vi "Scott -- strain -- manipulate sweep parameters V0.vi"(7 "sweep parameters action":T3, 10 "strain sweep control":T1={"just in case"=TRUE, "Piezo Amplifier settings"={"Gain "=69.44, "offset (V)"=69.44}, "voltage-parameters-IN"={"phase "=2.88, "amplitude (V)"=-0.7854, "offset (V)"=0.28, "time delay (sec)"=0.5, "period (sec)"=50.0, "shape"=enum."triangle"}, "Lockin Settings"=[{"Offset"=FALSE, "GPIB Address"=6}, {"Offset"=TRUE, "GPIB Address"=7}], "VISA address Agilent  IN"="GPIB0::22::INSTR", "number of iterations"=1.0, "Piezo sweep settings"={"max Piezo voltage (V) "=69.44, "min Piezo voltage (V)"=69.44, "delay (sec)"=69.44, "period (sec)"=69.44, "shape"=enum."triangle"}}) -> (2 "strain sweep control OUT":T1={"just in case"=TRUE, "Piezo Amplifier settings"={"Gain "=69.44, "offset (V)"=69.44}, "voltage-parameters-IN"={"phase "=2.88, "amplitude (V)"=-0.7854, "offset (V)"=0.28, "time delay (sec)"=0.5, "period (sec)"=50.0, "shape"=enum."triangle"}, "Lockin Settings"=[{"Offset"=FALSE, "GPIB Address"=6}, {"Offset"=TRUE, "GPIB Address"=7}], "VISA address Agilent  IN"="", "number of iterations"=1.0, "Piezo sweep settings"={"max Piezo voltage (V) "=69.44, "min Piezo voltage (V)"=69.44, "delay (sec)"=69.44, "period (sec)"=69.44, "shape"=enum."triangle"}})   [LabVIEW 2014]
uses:
  Scott -- strain -- strain sweep control.ctl
  FSU/ScottRiggs/Piezo2/voltage-wave-generator-parameters.ctl
  Scott -- strain -- sweep parameter action.ctl
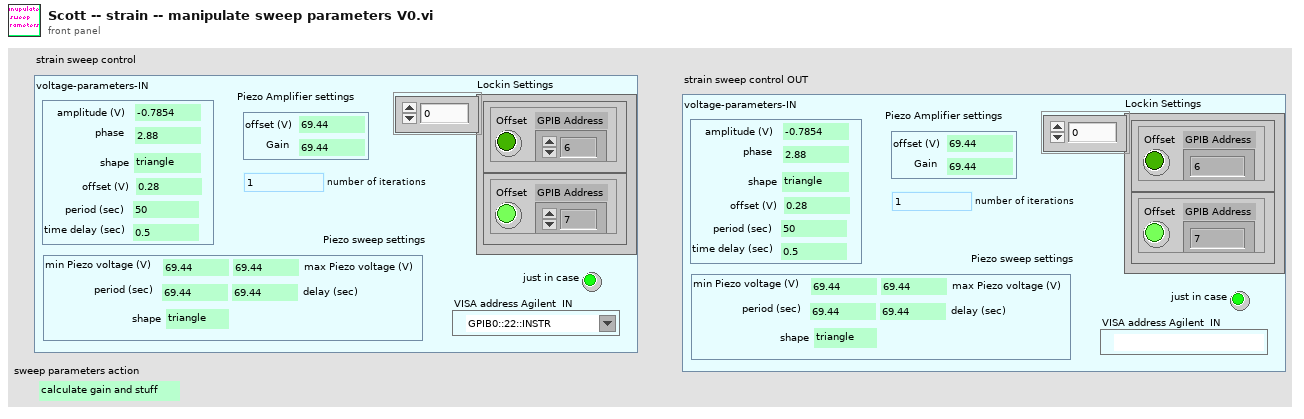
[diagram p1: front panel]
types:
  T1 = typedef "Scott -- strain -- strain sweep control.ctl" = cluster{"just in case":bool, "Piezo Amplifier settings":cluster{"Gain ":dbl, "offset (V)":dbl}, "voltage-parameters-IN":T2, "Lockin Settings":cluster{"Offset":bool, "GPIB Address":i16}[], "VISA address Agilent  IN":refnum<visa-resource-name>, "number of iterations":dbl, "Piezo sweep settings":cluster{"max Piezo voltage (V) ":dbl, "min Piezo voltage (V)":dbl, "delay (sec)":dbl, "period (sec)":dbl, "shape":enum16{"triangle", "sine", "none"}}}
  T2 = typedef "voltage-wave-generator-parameters.ctl" = cluster{"phase ":dbl, "amplitude (V)":dbl, "offset (V)":dbl, "time delay (sec)":dbl, "period (sec)":dbl, "shape":enum16{"triangle", "sine", "none"}}
  T3 = typedef "Scott -- strain -- sweep parameter action.ctl" = enum16{"calculate gain and stuff", "none"}
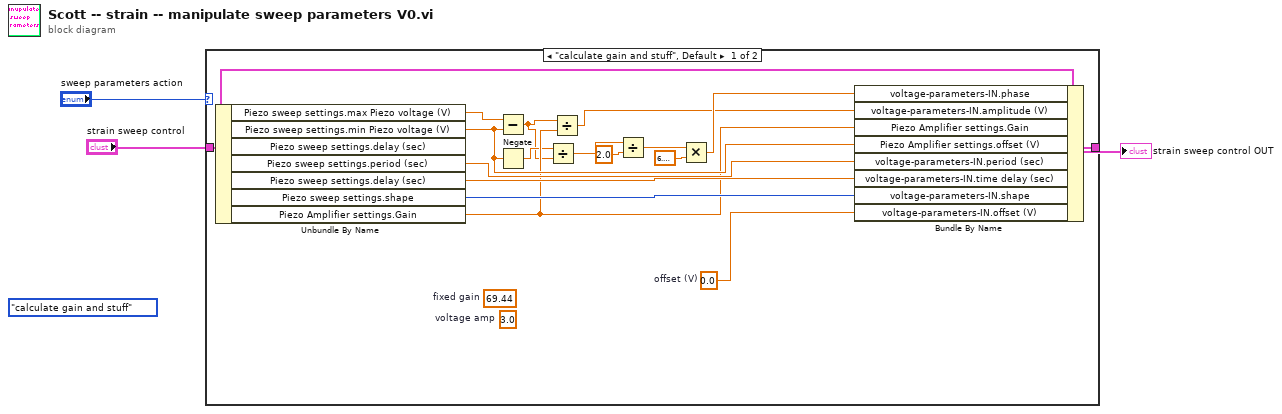
[diagram p0: block diagram]
diagram:
  (unwired) Scott_--_strain_--_sweep_parameter_action."calculate gain and stuff" ("sweep parameters action")
  n1 = case shown="\"calculate gain and stuff\", Default" "sweep parameters action" {
    tunnel: [w9 w21] -> w2
    tunnel: "strain sweep control" -> [w19 w21]
    frame "calculate gain and stuff", Default {
      (unwired) 69.44  # fixed gain
      w8 = 0.0  # offset (V)
      (unwired) 3.0  # voltage amp
      n2 = Unbundle By Name(w19) -> ("Piezo sweep settings.max Piezo voltage (V)"=w20:dbl, "Piezo sweep settings.min Piezo voltage (V)"=w18:dbl, "Piezo sweep settings.period (sec)"=w12:dbl, "Piezo sweep settings.delay (sec)"=w11:dbl, "Piezo sweep settings.shape"=w10:enum16{"triangle", "sine", "none"}, "Piezo Amplifier settings.Gain"=w7:dbl)  [unwired: 1 out]
      n3 = Subtract(x=w20, y=w18) -> (x-y=w4:dbl)
      n4 = Negate(x=w18) -> (-x=w5:dbl)
      n5 = Divide(x=w5, y=w4) -> (x/y=w17:dbl)
      n6 = Divide(x=w4, y=w7) -> (x/y=w6:dbl)
      n7 = Divide(x=w17, y=2.0) -> (x/y=w15:dbl)
      n8 = Multiply(x=w15, y=6.283185307179586) -> (x*y=w13:dbl)
      n9 = Bundle By Name(cluster=w19, "voltage-parameters-IN.phase"=w13, "voltage-parameters-IN.amplitude (V)"=w6, "Piezo Amplifier settings.Gain"=w7, "Piezo Amplifier settings.offset (V)"=w18, "voltage-parameters-IN.period (sec)"=w12, "voltage-parameters-IN.time delay (sec)"=w11, "voltage-parameters-IN.shape"=w10, "voltage-parameters-IN.offset (V)"=w8) -> (w9:T1)
    }
    frame "none" {
    }
  }
  "strain sweep control OUT" <- w2
